vi "Get Units.vi"(4 "error in":errorcluster caption="error in (no error)", 7 "VISA resource name in":refnum<visa-resource-name>) -> (0 "Fehler (Ausgang)":errorcluster caption="error out", 1 "PressureUnit":enum16{"bar", "psi"}(ring), 2 "TempUnit":enum16{"°C", "°F"}(ring), 3 "VISA resource name out":refnum<visa-resource-name>)   [LabVIEW 2015, in "JULABO DeviceDriver.lvlib"]
doc: "This VI returns the actual temperature unit (°C/°F) and pressure unit (bar/psi) of the device.\n\nNote:\nThis function is only available for Hightech-Circulators HL/SL. In case of °F, all temperatures are adjusted / returned in °F. Please use this VI to check whether the temperatures have to be adjusted in °C or in °F. Use this VI to check the unit of the return value of <B>Get Analog Pressure.vi</B>.\n\nThe temperature unit is not adjustable via this driver. Please adjust the temperature unit in the menu of your instrument (see operating manual)."
uses:
  JULABO DeviceDriver.lvlib
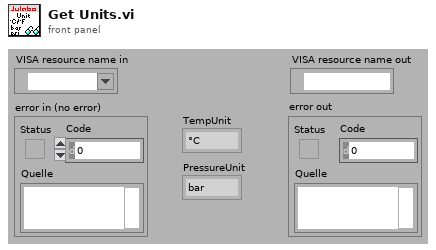
[diagram p1: front panel]
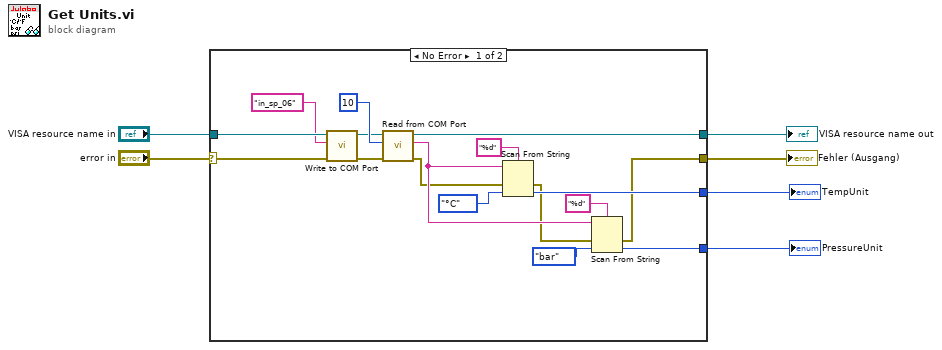
[diagram p0: block diagram]
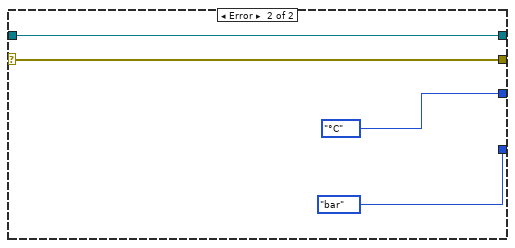
[diagram p2: hidden frame]
diagram:
  n1 = case shown="No Error" "error in" {
    selector: "error in" -> [w21 w26]
    tunnel: [w23 w27] -> w4
    tunnel: [w7 w26] -> w3
    tunnel: "VISA resource name in" -> [w22 w27]
    tunnel: [w15 enum16{"°C", "°F"}."°C" ("Enum")] -> w2
    tunnel: [w11 enum16{"bar", "psi"}."bar" ("PressureUnit")] -> w1
    frame No Error {
      n2 = call "Write to COM Port.vi"("error in"=w21, "Command (input)"="in_sp_06" ("Schreibpuffer"), "VISA resource name in"=w22) -> ("error out"=w17:errorcluster, "VISA resource name out"=w18:refnum<visa-resource-name>)  [unwired: 7 in]
      n3 = call "Read from COM Port.vi"("error in"=w17, "Byte to Read (-1:All)"=u32 10 ("Anzahl der Byte"), "VISA resource name in"=w18) -> ("error out"=w8:errorcluster, "String (output)"=w12:string, "VISA resource name out"=w23:refnum<visa-resource-name>)  [unwired: 5 in, 1 out]
      n4 = Scan From String(format string="%d" ("Format-String"), input string=w12, error in=w8, default 1=enum16{"°C", "°F"}."°C" ("Enum")) -> (error out=w9:errorcluster, output 1=w15:enum16{"°C", "°F"})  [unwired: 1 in, 2 out]
      n5 = Scan From String(format string="%d" ("Format-String"), input string=w12, error in=w9, default 1=enum16{"bar", "psi"}."bar" ("PressureUnit")) -> (error out=w7:errorcluster, output 1=w11:enum16{"bar", "psi"})  [unwired: 1 in, 2 out]
    }
    frame Error {
    }
  }
  "Fehler (Ausgang)" <- w3
  "VISA resource name out" <- w4
  "TempUnit" <- w2
  "PressureUnit" <- w1
